vi "Actor Core.vi"(8 "error in":errorcluster, 11 "Commissioning in":refnum<class "Commissioning.lvclass">) -> (0 "error out":errorcluster, 3 "Actor out":refnum<class "Actor.lvclass">)   [LabVIEW 2018, in "Commissioning Actor.lvlib" / "Commissioning.lvclass"]
doc: "(<B>Filename</B>: Actor Framework.lvlib:Actor.lvclass:Actor Core.vi)\n\nReceives messages to the actor, reacts to them, and initiates any error handling that may shut the actor down.\n\nDescendant classes may override this VI to append parallel tasks for the actor to complete while it handles messages. Overrides use the Call Parent Method node."
uses:
  Commissioning.lvclass
  C:/Users/Administrator/Desktop/LabVIEW EMS/EMS Generic Actor/EMS Generic/EMS Generic.lvclass
  C:/Users/Administrator/Desktop/LabVIEW EMS/Device Communication and Control Abstract Actor/Device Communication and Control Abstract/Device Communication and Control Abstract.lvclass
  C:/Program Files (x86)/National Instruments/LabVIEW 2018/vi.lib/ActorFramework/Actor/Actor.lvclass
  <vilib>/ActorFramework/Actor/Actor.lvclass
  <vilib>/ORNL/CSEISMIC DDS/CSEISMIC DDS Base/Data Types/Controls/DeviceID.ctl
  EMS Generic Actor/EMS Generic/EMS Generic.lvclass/EMS Generic.ctl
  <vilib>/ORNL/CSEISMIC DDS/CSEISMIC DDS Base/Data Types/Controls/DeviceClass Selector.ctl
  <vilib>/ActorFramework/Actor/Actor.lvclass/Actor.ctl
  Device Communication and Control Abstract Actor/Device Communication and Control Abstract/Device Communication and Control Abstract.lvclass/Device Communication and Control Abstract.ctl
  <vilib>/ActorFramework/Message Enqueuer/Message Enqueuer.lvclass/Message Enqueuer.ctl
  Commissioning.lvclass/Commissioning.ctl
  Controls/Activate or Blackstart Selector.ctl
  Commissioning Messages/Activate or Blackstart Msg/Activate or Blackstart Msg.lvclass/Activate or Blackstart Msg.ctl
  <vilib>/ORNL/CSEISMIC DDS/CSEISMIC DDS Base/Data Types/DER_Measurement.ctl
  <vilib>/ORNL/CSEISMIC DDS/CSEISMIC DDS Base/Data Types/DER_Info.ctl
  <vilib>/ORNL/CSEISMIC DDS/CSEISMIC DDS Base/Data Types/Meter_Measurement.ctl
  <vilib>/ORNL/CSEISMIC DDS/CSEISMIC DDS Base/Data Types/Meter_Info.ctl
  <vilib>/ORNL/CSEISMIC DDS/CSEISMIC DDS Base/Data Types/SmartRelay_Measurement.ctl
  <vilib>/ORNL/CSEISMIC DDS/CSEISMIC DDS Base/Data Types/SmartRelay_Info.ctl
  <vilib>/ActorFramework/Message Enqueuer/Enqueue.vi
  EMS Generic Actor/EMS Generic/Accessors - Global Configuration/Read Global Configuration.vi
  Device Communication and Control Abstract Actor/Device Communication and Control Abstract Messages/Set IED MicrogridID Msg/Set IED MicrogridID Msg.lvclass
  C:/Program Files (x86)/National Instruments/LabVIEW 2018/vi.lib/ActorFramework/Message/Message.lvclass
  Commissioning Messages/Activate or Blackstart Msg/Activate or Blackstart Msg.lvclass
  <vilib>/ActorFramework/Message Priority Queue/Priority Enqueue.vi
  EMS Generic Actor/EMS Generic/Accessors - Global Configuration/Update Global Configuration.vi
  Generic Optimization Actor/Generic Optimization/Generic Optimization.lvclass
  Device Communication and Control Abstract Actor/Device Communication and Control Abstract/Device Communication and Control Abstract.lvclass
  EMS Generic Actor/EMS Generic/EMS Generic.lvclass
  <vilib>/ORNL/CSEISMIC DDS/CSEISMIC DDS Base/CSEISMIC DDS.lvclass
  Global Variables/Global Variables.vi
panel:
  out "PrimaryVoltage":dbl[](array[numeric])
  out "PCC DeviceID":T1
  out "Low Voltage":dbl
  out "High Voltage":dbl
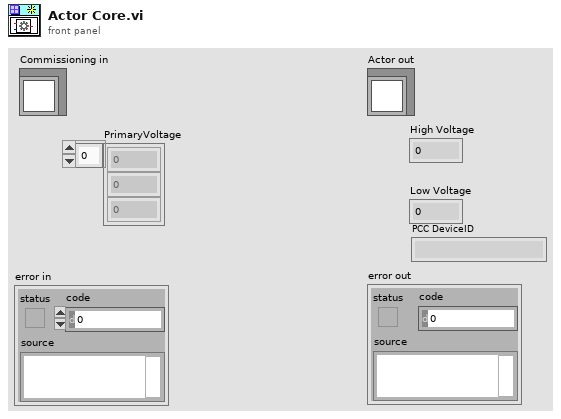
[diagram p1: front panel]
types:
  T1 = typedef "CSEISMIC DDS.lvlib/CSEISMIC DDS.lvclass/DeviceID.ctl" = string
  T2 = enum32{"Invalid", "Standard", "Closed", "Hidden", "Minimized", "Maximized"}
  T3 = typedef "EMS Generic Actor.lvlib/EMS Generic.lvclass/Data Type DVRs.ctl" = cluster{"IED_Status":refnum<data-value>, "IED_Status_0":refnum<data-value>, "DER_Measurement":refnum<data-value>, "DER_Info":refnum<data-value>, "DER_Status":refnum<data-value>, "ES_Measurement":refnum<data-value>, "ES_Info":refnum<data-value>, "PV_Info":refnum<data-value>, "SmartRelay_Info":refnum<data-value>, "SmartRelay_Measurement":refnum<data-value>, "Meter_Info":refnum<data-value>, "Meter_Measurement":refnum<data-value>, "HVAC_Status":refnum<data-value>, "HVAC_Measurement":refnum<data-value>, "PriceData_RealTime":refnum<data-value>, "PriceData_Demand":refnum<data-value>, "PriceData_Energy":refnum<data-value>, "ForecastData_Long":refnum<data-value>, "ForecastData_Short":refnum<data-value>, "DER_Control":refnum<data-value>, "DER_SetPointF":refnum<data-value>, "DER_SetPointP":refnum<data-value>, "DER_SetPointQ":refnum<data-value>, "DER_SetPointPF":refnum<data-value>, "DER_SetPointV":refnum<data-value>, "PV_setCurtailment":refnum<data-value>, "PV_setRampRate":refnum<data-value>, "Relay_Control":refnum<data-value>, "Load_Control":refnum<data-value>, "HVAC_Control":refnum<data-value>, "Generator_Info":refnum<data-value>, "ForecastData_Long_Backup":refnum<data-value>, "PriceData_RealTime_Backup":refnum<data-value>}
  T4 = typedef "CSEISMIC DDS.lvlib/CSEISMIC DDS.lvclass/DeviceClass Selector.ctl" = u16
  T5 = typedef "Commissioning Actor.lvlib/Commissioning.lvclass/Activate or Blackstart Selector.ctl" = enum16{"Activate", "Blackstart"}
  T6 = typedef "CSEISMIC DDS.lvlib/CSEISMIC DDS.lvclass/Meter_Info.ctl" = cluster{"DeviceID":T1, "LineConfig":u8[], "NominalVoltage(V)":dbl}
  T7 = typedef "CSEISMIC DDS.lvlib/CSEISMIC DDS.lvclass/Meter_Measurement.ctl" = cluster{"DeviceID":T1, "Voltage":dbl[], "Current":dbl[], "RealPower":dbl[], "ReactivePower":dbl[], "LineConfig":u8[], "Frequency":dbl}
  T8 = typedef "CSEISMIC DDS.lvlib/CSEISMIC DDS.lvclass/DER_Info.ctl" = cluster{"DeviceID":T1, "LineConfig":u8[], "NominalVoltage(V)":dbl, "PowerRating(kVA)":dbl, "VFControl":bool, "PControl":bool, "QControl":bool, "PFControl":bool, "PVControl":bool, "Droop":bool, "DroopConfigurable":bool, "Unbalanced":bool}
  T9 = typedef "CSEISMIC DDS.lvlib/CSEISMIC DDS.lvclass/DER_Measurement.ctl" = cluster{"DeviceID":T1, "Voltage":dbl[], "Current":dbl[], "RealPower":dbl[], "ReactivePower":dbl[], "LineConfig":u8[], "Frequency":dbl}
  T10 = typedef "CSEISMIC DDS.lvlib/CSEISMIC DDS.lvclass/SmartRelay_Info.ctl" = cluster{"DeviceID":T1, "LineConfig":u8[], "NominalVoltage(V)":dbl}
  T11 = typedef "CSEISMIC DDS.lvlib/CSEISMIC DDS.lvclass/SmartRelay_Measurement.ctl" = cluster{"DeviceID":T1, "PrimaryVoltage":dbl[], "SecondaryVoltage":dbl[], "Current":dbl[], "RealPower":dbl[], "ReactivePower":dbl[], "LineConfig":u8[], "Frequency":dbl}
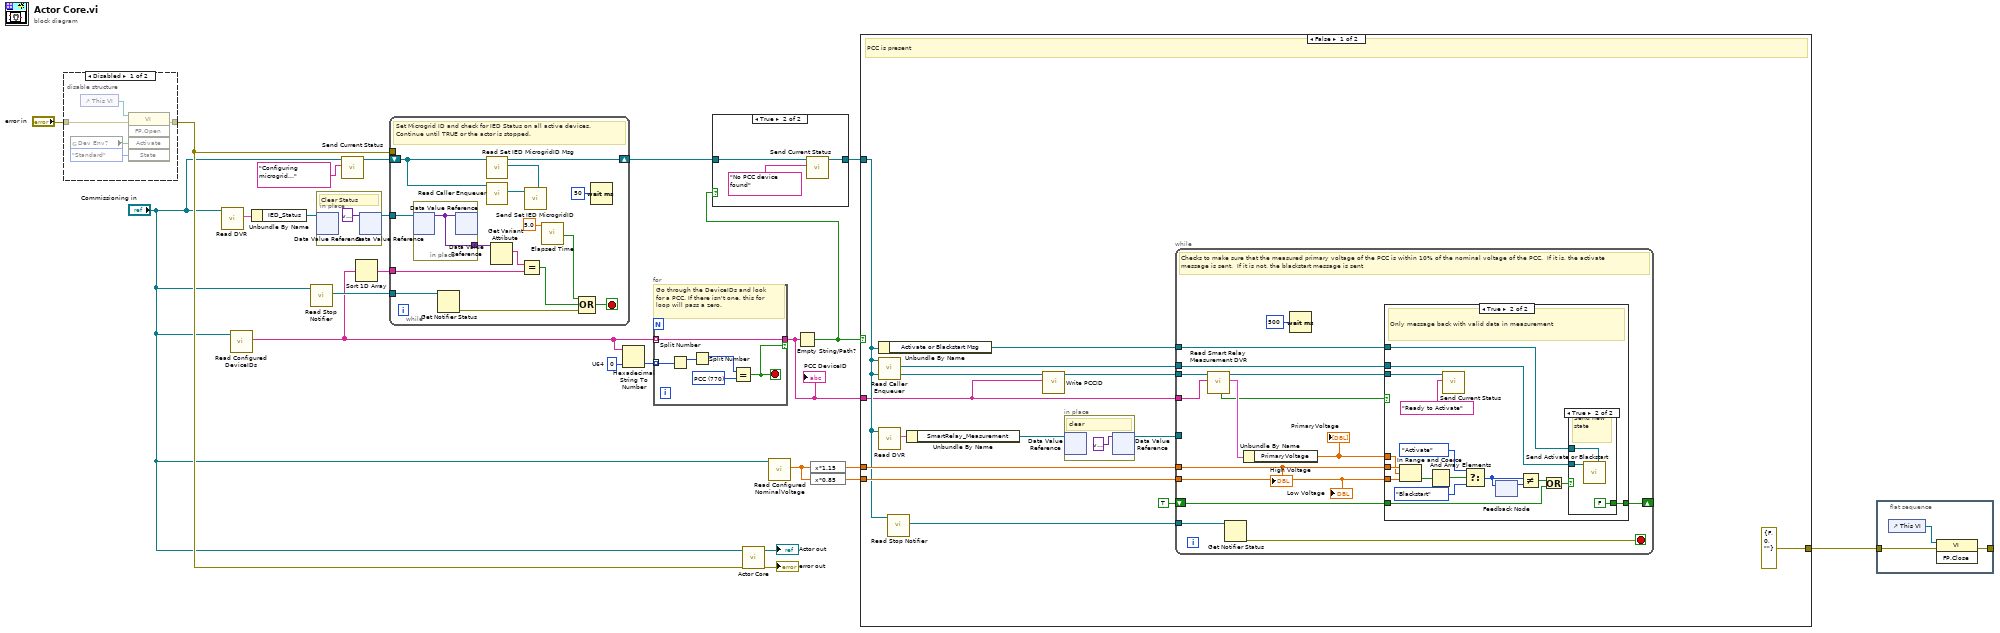
[diagram p0: block diagram]
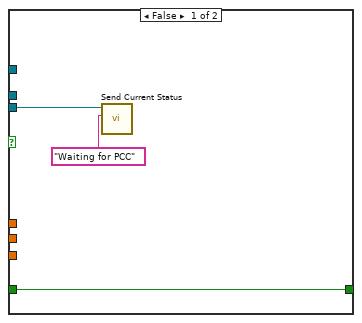
[diagram p4: hidden frame]
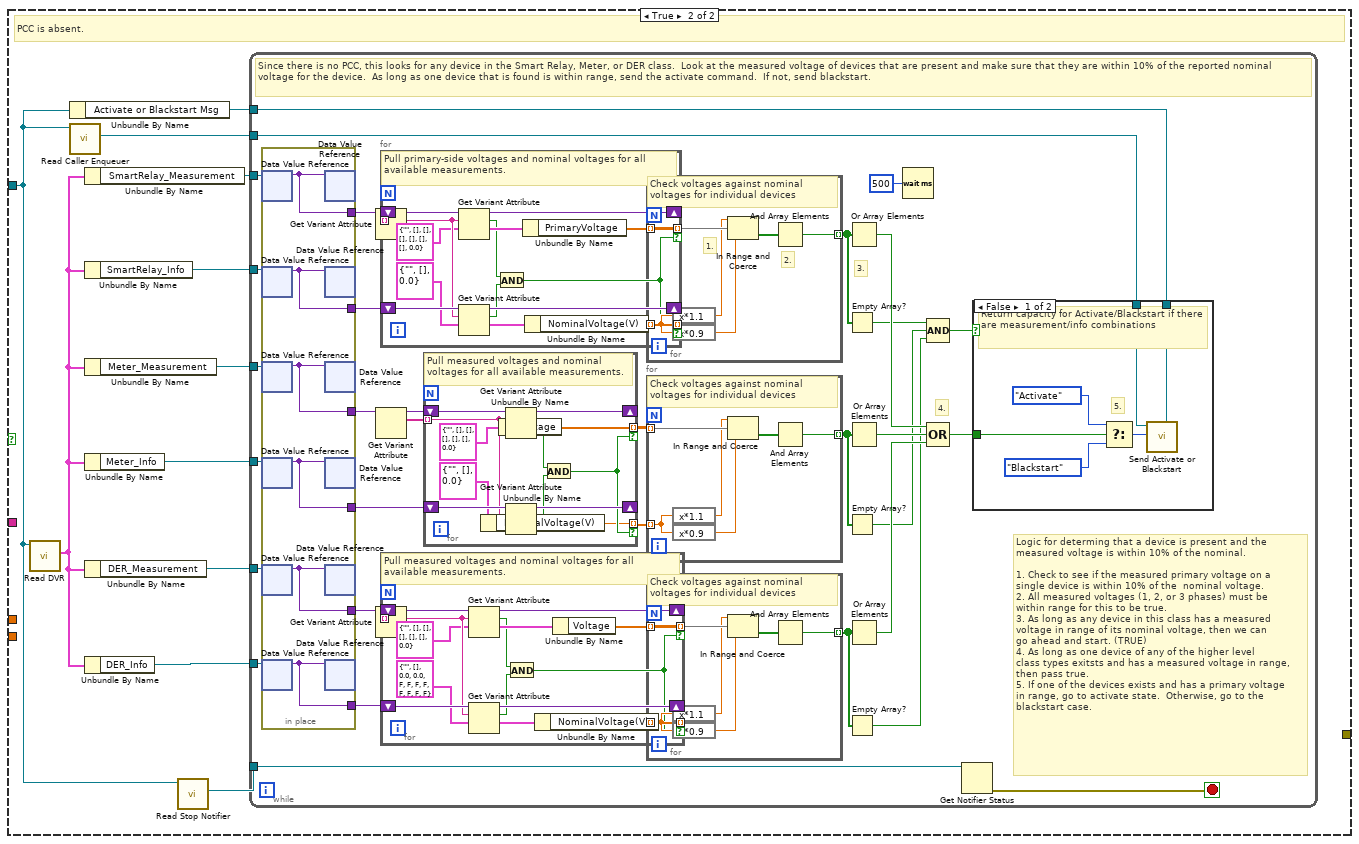
[diagram p6: hidden frame]
diagram:
  w15 = u64 0  # U64
  n1 = disable-structure shown="Disabled" {
    disable-tunnel: "error in" -> [w26 w29]
    disable-tunnel: [w25 w29] -> w10
    frame Disabled {
      n2 = global read "Global Variables.vi" "Dev Env?"() -> (w24:bool)
      n3 = control-ref of="This VI"() -> (w28:refnum<vi>)
      n4 = invoke class="VI" method="FP.Open"(reference=w28, error in=w26, "Activate"=w24, "State"=T2."Standard") -> (error out=w25:errorcluster)  [unwired: 1 in, 4 out]
    }
    frame Enabled {
    }
  }
  n5 = call "Read DVR.vi"("EMS Generic in"="Commissioning in") -> ("DVR"=w19:T3)  [unwired: 9 in, 1 out]
  n6 = call "Read Configured DeviceIDs.vi"("EMS Generic in"="Commissioning in") -> ("DeviceIDs"=w9:T1[])  [unwired: 8 in, 2 out]
  n7 = Unbundle By Name(w19) -> ("IED_Status"=w14:refnum<data-value>)
  n8 = call "Read Stop Notifier.vi"("EMS Generic in"="Commissioning in") -> ("stop"=w16:refnum<notifier>)  [unwired: 9 in, 1 out]
  n9 = in-place {
    # "Clear Status"
    n10 = in-place-dvr #1(w14) -> ()  [unwired: 2 out]
    n11 = in-place-dvr #1(variant ("data value")) -> (w13:refnum<data-value>)  [unwired: 1 out]
  }
  n12 = call "Send Current Status.vi"("Current Status"="Configuring microgrid...", "Device Communication and Control Abstract in"="Commissioning in") -> ("Device Communication and Control Abstract out"=w5:refnum<class "Commissioning.lvclass">)  [unwired: 8 in, 1 out]
  n13 = Sort 1D Array(array=w9) -> (sorted array=w8:T1[])
  n14 = while {
    tunnel: w13 -> [w41]
    tunnel: w16 -> [w45]
    shift-right: [w38] -> w3
    shift-left: w5 -> [w36]
    tunnel: w10 -> [_]
    tunnel: w8 -> [w33]
    stop <- w39 stop-if-true
    # "Set Microgrid ID and check for IED Status on all active devices. Continue until TRUE or the actor is stopped."
    n15 = in-place {
      in-place-border: [w46] -> w42
      n16 = in-place-dvr #2(w41) -> (w46:variant)  [unwired: 1 out]
      n17 = in-place-dvr #2(w46) -> ()  [unwired: 2 out]
    }
    n18 = Get Notifier Status(notifier=w45) -> (error out=w40:errorcluster)  [unwired: 1 in, 4 out]
    n19 = call "Read Set IED MicrogridID Msg.vi"("SCADA Sub Abstract in"=w36) -> ("Set IED MicrogridID Msg"=w43:refnum<class "Set IED MicrogridID Msg.lvclass">, "SCADA Sub Abstract out"=w38:refnum<class "Commissioning.lvclass">)  [unwired: 9 in]
    n20 = call <vilib>:"Read Caller Enqueuer.vi"("Actor"=w36) -> ("Caller Enqueuer"=w44:refnum<class "Message Enqueuer.lvclass">)  [unwired: 10 in]
    n21 = Get Variant Attribute(Variant=w42) -> (names=w35:string[])  [unwired: 3 in, 3 out]
    n22 = Equal?(x=w35, y=w33) -> (x = y?=w34:bool)
    n23 = call "Send Set IED MicrogridID.vi"("Message Type"=w43, "Message Enqueuer"=w44) -> ()  [unwired: 8 in, 2 out]
    n24 = call "Elapsed Time"("Time Target (s)"=5.0) -> ("Time has Elapsed"=w31:bool)  [unwired: 11 in, 7 out]
    n25 = Compound Arithmetic op=OR(w31, w34, w40) -> (w39:bool)
    n26 = Wait (ms)(milliseconds to wait=u32 50) -> ()  [unwired: 1 out]
  }
  n27 = Hexadecimal String To Number(string=w9, default (0uL)=w15) -> (number=w18:u64[])  [unwired: 1 in, 1 out]
  n28 = for {
    tunnel: w9 -> [w51] mode=indexing
    tunnel: [w51] -> w22 if=w48
    tunnel: w18 -> [w47] mode=indexing
    stop <- w48 stop-if-true
    w50 = T4 770 items=["Invalid"=0, "IED"=256, "DER"=512, "Relay"=768, "Meter"=1024, "Load"=1280, "Energy Storage"=513, "PV"=514, "Generator"=515, "Smart Relay"=769, "PCC"=770, "Smart Meter"=1025, "PMU"=1026, "HVAC"=1281] ("DeviceClass")
    # "Go through the DeviceIDs and look for a PCC. If there isn't one, this for loop will pass a zero."
    n29 = Split Number(x=w47) -> (hi(x)=w52:u32)  [unwired: 1 out]
    n30 = Split Number(x=w52) -> (hi(x)=w49:u16)  [unwired: 1 out]
    n31 = Equal?(x=w49, y=w50) -> (x = y?=w48:bool)
  }
  "PCC DeviceID" <- w22
  n32 = call-parent "Actor Core.vi"("error in"=w10, "Actor in"="Commissioning in") -> ("error out"=→"error out":errorcluster, "Actor out"=→"Actor out":refnum<class "Actor.lvclass">)  [unwired: 8 in]
  n33 = call "Read Configured NominalVoltage.vi"("EMS Generic in"="Commissioning in") -> ("NominalVoltage"=w7:dbl)  [unwired: 8 in, 2 out]
  n34 = Empty String/Path?(string/path=w22) -> (empty?=w1:bool)
  n35 = case shown="True" w1 {
    tunnel: w3 -> [w53 w55]
    tunnel: [w53 w54] -> w2
    frame False {
    }
    frame True {
      n36 = call "Send Current Status.vi"("Current Status"="No PCC device found", "Device Communication and Control Abstract in"=w55) -> ("Device Communication and Control Abstract out"=w54:refnum<class "Commissioning.lvclass">)  [unwired: 8 in, 1 out]
    }
  }
  n37 = expression code="x*1.15"(w7) -> (w21:dbl)
  n38 = expression code="x*0.85"(w7) -> (w20:dbl)
  n39 = case shown="False" w1 {
    tunnel: w22 -> [w59 _]
    tunnel: w2 -> [w60 w109]
    tunnel: w21 -> [w68 _]
    tunnel: w20 -> [w67 _]
    tunnel: [errorcluster {"status"=FALSE, "code"=0, "source"=""} ("error in (no error)") _] -> w12
    frame False {
      # "PCC is present"
      n40 = Unbundle By Name(w60) -> ("Activate or Blackstart Msg"=w65:refnum<class "Activate or Blackstart Msg.lvclass">)
      n41 = call <vilib>:"Read Caller Enqueuer.vi"("Actor"=w60) -> ("Caller Enqueuer"=w66:refnum<class "Message Enqueuer.lvclass">)  [unwired: 10 in]
      n42 = call "Read DVR.vi"("EMS Generic in"=w60) -> ("DVR"=w69:T3)  [unwired: 9 in, 1 out]
      n43 = call "Read Stop Notifier.vi"("EMS Generic in"=w60) -> ("stop"=w64:refnum<notifier>)  [unwired: 9 in, 1 out]
      n44 = Unbundle By Name(w69) -> ("SmartRelay_Measurement"=w63:refnum<data-value>)
      n45 = call "Write PCCID.vi"("PCCID"=w59, "EMS Generic in"=w60) -> ("EMS Generic out"=w58:refnum<class "Commissioning.lvclass">)  [unwired: 8 in, 1 out]
      n46 = in-place {
        # "clear"
        n47 = in-place-dvr #3(w63) -> ()  [unwired: 2 out]
        n48 = in-place-dvr #3(variant ("data value")) -> (w62:refnum<data-value>)  [unwired: 1 out]
      }
      n49 = while {
        tunnel: w62 -> [_]
        tunnel: w59 -> [w76]
        tunnel: w68 -> [w85]
        tunnel: w67 -> [w84]
        tunnel: w66 -> [w82]
        tunnel: w65 -> [w81]
        tunnel: w64 -> [w80]
        tunnel: w58 -> [w77]
        shift-right: [w71] -> _
        shift-left: TRUE -> [w72]
        stop <- w79 stop-if-true
        # "Checks to make sure that the measured primary voltage of the PCC is within 10% of the nominal voltage of the PCC.  If it is, the activate message is sent.  If it is not, the blackstart message is sent"
        n50 = call "Read Smart Relay Measurement DVR.vi"("DeviceID"=w76, "EMS Generic in"=w77) -> ("SmartRelay_Measurement"=w75:T11, "EMS Generic out"=w73:refnum<class "Commissioning.lvclass">, "valid?"=w74:bool)  [unwired: 6 in, 1 out]
        n51 = Get Notifier Status(notifier=w80) -> (error out=w79:errorcluster)  [unwired: 1 in, 4 out]
        n52 = Unbundle By Name(w75) -> ("PrimaryVoltage"=w83:dbl[])
        "PrimaryVoltage" <- w83
        n53 = Wait (ms)(milliseconds to wait=u32 500) -> ()  [unwired: 1 out]
        n54 = case shown="True" w74 {
          tunnel: w85 -> [_ w105]
          tunnel: w84 -> [_ w104]
          tunnel: w83 -> [_ w103]
          tunnel: w82 -> [_ w101]
          tunnel: w81 -> [_ w100]
          tunnel: w73 -> [w87 w95]
          tunnel: w72 -> [w86 w90]
          tunnel: [w86 w89] -> w71
          frame False {
            n55 = call "Send Current Status.vi"("Current Status"="Waiting for PCC", "Device Communication and Control Abstract in"=w87) -> ()  [unwired: 8 in, 2 out]
          }
          frame True {
            # "Only message back with valid data in measurement"
            n56 = In Range and Coerce(upper limit=w105, x=w103, lower limit=w104) -> (In Range?=w102:bool[])  [unwired: 1 out]
            n57 = And Array Elements(Boolean array=w102) -> (logical AND=w99:bool)
            n58 = call "Send Current Status.vi"("Current Status"="Ready to Activate", "Device Communication and Control Abstract in"=w95) -> ()  [unwired: 8 in, 2 out]
            n59 = Select(t=Activate_or_Blackstart_Selector."Activate" ("Activate or Blackstart"), s=w99, f=Activate_or_Blackstart_Selector."Blackstart" ("Activate or Blackstart")) -> (s? t:f=w93:T5)
            n60 = feedback-in #4(w93) -> ()
            n61 = feedback #4() -> (w94:T5)  [unwired: 1 in]
            n62 = Not Equal?(x=w93, y=w94) -> (x != y?=w92:bool)
            n63 = Or(x=w92, y=w90) -> (x .or. y?=w91:bool)
            n64 = case shown="True" w91 {
              tunnel: w101 -> [_ w108]
              tunnel: w100 -> [_ w107]
              tunnel: [_ FALSE] -> w89
              frame False {
                # "Already sent this message.  Do nothing."
              }
              frame True {
                # "Send new state"
                n65 = call "Send Activate or Blackstart.vi"("Message Type"=w107, "Message Enqueuer"=w108) -> ()  [unwired: 8 in, 2 out]
              }
            }
          }
        }
        "High Voltage" <- w85
        "Low Voltage" <- w84
      }
    }
    frame True {
      # "PCC is absent."
      n66 = call "Read DVR.vi"("EMS Generic in"=w109) -> ("DVR"=w111:T3)  [unwired: 9 in, 1 out]
      n67 = Unbundle By Name(w109) -> ("Activate or Blackstart Msg"=w113:refnum<class "Activate or Blackstart Msg.lvclass">)
      n68 = call <vilib>:"Read Caller Enqueuer.vi"("Actor"=w109) -> ("Caller Enqueuer"=w112:refnum<class "Message Enqueuer.lvclass">)  [unwired: 10 in]
      n69 = Unbundle By Name(w111) -> ("SmartRelay_Measurement"=w114:refnum<data-value>)
      n70 = Unbundle By Name(w111) -> ("SmartRelay_Info"=w115:refnum<data-value>)
      n71 = Unbundle By Name(w111) -> ("Meter_Measurement"=w116:refnum<data-value>)
      n72 = Unbundle By Name(w111) -> ("Meter_Info"=w118:refnum<data-value>)
      n73 = Unbundle By Name(w111) -> ("DER_Measurement"=w117:refnum<data-value>)
      n74 = Unbundle By Name(w111) -> ("DER_Info"=w119:refnum<data-value>)
      n75 = call "Read Stop Notifier.vi"("EMS Generic in"=w109) -> ("stop"=w110:refnum<notifier>)  [unwired: 9 in, 1 out]
      n76 = while {
        tunnel: w119 -> [w159]
        tunnel: w118 -> [w158]
        tunnel: w117 -> [w157]
        tunnel: w116 -> [w156]
        tunnel: w115 -> [w155]
        tunnel: w114 -> [w154]
        tunnel: w113 -> [w131]
        tunnel: w112 -> [w121]
        tunnel: w110 -> [w130]
        stop <- w129 stop-if-true
        # "Logic for determing that a device is present and the\nmeasured voltage is within 10% of the nominal.\n\n1. Check to see if the measured primary voltage on a\nsingle device is within 10% of the  nominal voltage.\n2. All measured voltages (1, 2, or 3 phases) must be \nwithin range for this to be true.\n3. As long as any device in this class has a measured\nvoltage in range of its nominal voltage, then we can\ngo ahead and start. (TRUE)\n4. As long as one device of any of the higher level \nclass types exitsts and has a measured voltage in range,\nthen pass true.\n5. If one of the devices exists and has a primary voltage\nin range, go to activate state.  Otherwise, go to the\nblackstart case."
        # "4."
        # "3."
        # "Since there is no PCC, this looks for any device in the Smart Relay, Meter, or DER class.  Look at the measured voltage of devices that are present and make sure that they are within 10% of the reported nominal voltage for the device.  As long as one device that is found is within range, send the activate command.  If not, send blackstart."
        n77 = in-place {
          in-place-border: [w179] -> w151
          in-place-border: [w178] -> w150
          in-place-border: [w177] -> w147
          in-place-border: [w176] -> w146
          in-place-border: [w175] -> w143
          in-place-border: [w174] -> w142
          n78 = in-place-dvr #5(w154) -> (w179:variant)  [unwired: 1 out]
          n79 = in-place-dvr #6(w155) -> (w178:variant)  [unwired: 1 out]
          n80 = in-place-dvr #7(w156) -> (w177:variant)  [unwired: 1 out]
          n81 = in-place-dvr #8(w158) -> (w176:variant)  [unwired: 1 out]
          n82 = in-place-dvr #9(w157) -> (w175:variant)  [unwired: 1 out]
          n83 = in-place-dvr #10(w159) -> (w174:variant)  [unwired: 1 out]
          n84 = in-place-dvr #5(w179) -> ()  [unwired: 2 out]
          n85 = in-place-dvr #6(w178) -> ()  [unwired: 2 out]
          n86 = in-place-dvr #7(w177) -> ()  [unwired: 2 out]
          n87 = in-place-dvr #8(w176) -> ()  [unwired: 2 out]
          n88 = in-place-dvr #9(w175) -> ()  [unwired: 2 out]
          n89 = in-place-dvr #10(w174) -> ()  [unwired: 2 out]
        }
        n90 = Get Variant Attribute(Variant=w151) -> (duplicate Variant=w152:variant, names=w153:string[])  [unwired: 3 in, 2 out]
        n91 = Get Variant Attribute(Variant=w147) -> (duplicate Variant=w149:variant, names=w148:string[])  [unwired: 3 in, 2 out]
        n92 = Get Variant Attribute(Variant=w143) -> (duplicate Variant=w144:variant, names=w145:string[])  [unwired: 3 in, 2 out]
        n93 = for {
          shift-right: [w206] -> _
          shift-left: w152 -> [w207]
          shift-right: [w204] -> _
          shift-left: w150 -> [w205]
          tunnel: w153 -> [w203] mode=indexing
          tunnel: [w195] -> w140 mode=indexing if=w196
          tunnel: [w194] -> w141 mode=indexing if=w196
          # "Pull primary-side voltages and nominal voltages for all available measurements."
          n94 = Get Variant Attribute(Variant=w207, name=w203, default value (empty Variant)=T11 {"DeviceID"="", "PrimaryVoltage"=[], "SecondaryVoltage"=[], "Current"=[], "RealPower"=[], "ReactivePower"=[], "LineConfig"=[], "Frequency"=0.0} ("SmartRelay_Measurement")) -> (duplicate Variant=w206:variant, found=w199:bool, value=w201:T11)  [unwired: 1 in, 1 out]
          n95 = Get Variant Attribute(Variant=w205, name=w203, default value (empty Variant)=T10 {"DeviceID"="", "LineConfig"=[], "NominalVoltage(V)"=0.0} ("SmartRelay_Info")) -> (duplicate Variant=w204:variant, found=w200:bool, value=w197:T10)  [unwired: 1 in, 1 out]
          n96 = And(x=w199, y=w200) -> (x .and. y?=w196:bool)
          n97 = Unbundle By Name(w201) -> ("PrimaryVoltage"=w195:dbl[])
          n98 = Unbundle By Name(w197) -> ("NominalVoltage(V)"=w194:dbl)
        }
        n99 = for {
          shift-right: [w192] -> _
          shift-left: w144 -> [w193]
          shift-right: [w190] -> _
          shift-left: w142 -> [w191]
          tunnel: w145 -> [w189] mode=indexing
          tunnel: [w183] -> w138 mode=indexing if=w184
          tunnel: [w182] -> w137 mode=indexing if=w184
          # "Pull measured voltages and nominal voltages for all available measurements."
          n100 = Get Variant Attribute(Variant=w193, name=w189, default value (empty Variant)=T9 {"DeviceID"="", "Voltage"=[], "Current"=[], "RealPower"=[], "ReactivePower"=[], "LineConfig"=[], "Frequency"=0.0} ("DER_Measurement")) -> (duplicate Variant=w192:variant, found=w186:bool, value=w188:T9)  [unwired: 1 in, 1 out]
          n101 = Get Variant Attribute(Variant=w191, name=w189, default value (empty Variant)=T8 {"DeviceID"="", "LineConfig"=[], "NominalVoltage(V)"=0.0, "PowerRating(kVA)"=0.0, "VFControl"=FALSE, "PControl"=FALSE, "QControl"=FALSE, "PFControl"=FALSE, "PVControl"=FALSE, "Droop"=FALSE, "DroopConfigurable"=FALSE, "Unbalanced"=FALSE} ("DER_Info")) -> (duplicate Variant=w190:variant, found=w187:bool, value=w185:T8)  [unwired: 1 in, 1 out]
          n102 = And(x=w186, y=w187) -> (x .and. y?=w184:bool)
          n103 = Unbundle By Name(w185) -> ("NominalVoltage(V)"=w182:dbl)
          n104 = Unbundle By Name(w188) -> ("Voltage"=w183:dbl[])
        }
        n105 = for {
          shift-right: [w172] -> _
          shift-left: w149 -> [w173]
          shift-right: [w170] -> _
          shift-left: w146 -> [w171]
          tunnel: w148 -> [w169] mode=indexing
          tunnel: [w163] -> w139 mode=indexing if=w164
          tunnel: [w162] -> w136 mode=indexing if=w164
          # "Pull measured voltages and nominal voltages for all available measurements."
          n106 = Get Variant Attribute(Variant=w173, name=w169, default value (empty Variant)=T7 {"DeviceID"="", "Voltage"=[], "Current"=[], "RealPower"=[], "ReactivePower"=[], "LineConfig"=[], "Frequency"=0.0} ("Meter_Measurement")) -> (duplicate Variant=w172:variant, found=w166:bool, value=w168:T7)  [unwired: 1 in, 1 out]
          n107 = Unbundle By Name(w168) -> ("Voltage"=w163:dbl[])
          n108 = Get Variant Attribute(Variant=w171, name=w169, default value (empty Variant)=T6 {"DeviceID"="", "LineConfig"=[], "NominalVoltage(V)"=0.0} ("Meter_Info")) -> (duplicate Variant=w170:variant, found=w167:bool, value=w165:T6)  [unwired: 1 in, 1 out]
          n109 = Unbundle By Name(w165) -> ("NominalVoltage(V)"=w162:dbl)
          n110 = And(x=w166, y=w167) -> (x .and. y?=w164:bool)
        }
        n111 = for {
          tunnel: w141 -> [w231] mode=indexing
          tunnel: w140 -> [w230] mode=indexing
          tunnel: [w226] -> w127 mode=indexing
          # "2."
          # "1."
          # "Check voltages against nominal voltages for individual devices"
          n112 = expression code="x*1.1"(w231) -> (w229:dbl)
          n113 = expression code="x*0.9"(w231) -> (w228:dbl)
          n114 = In Range and Coerce(upper limit=w229, x=w230, lower limit=w228) -> (In Range?=w227:bool[])  [unwired: 1 out]
          n115 = And Array Elements(Boolean array=w227) -> (logical AND=w226:bool)
        }
        n116 = for {
          tunnel: w136 -> [w225] mode=indexing
          tunnel: w139 -> [w224] mode=indexing
          tunnel: [w220] -> w126 mode=indexing
          # "Check voltages against nominal voltages for individual devices"
          n117 = expression code="x*1.1"(w225) -> (w223:dbl)
          n118 = expression code="x*0.9"(w225) -> (w222:dbl)
          n119 = In Range and Coerce(upper limit=w223, x=w224, lower limit=w222) -> (In Range?=w221:bool[])  [unwired: 1 out]
          n120 = And Array Elements(Boolean array=w221) -> (logical AND=w220:bool)
        }
        n121 = for {
          tunnel: w137 -> [w219] mode=indexing
          tunnel: w138 -> [w218] mode=indexing
          tunnel: [w214] -> w125 mode=indexing
          # "Check voltages against nominal voltages for individual devices"
          n122 = expression code="x*1.1"(w219) -> (w217:dbl)
          n123 = expression code="x*0.9"(w219) -> (w216:dbl)
          n124 = In Range and Coerce(upper limit=w217, x=w218, lower limit=w216) -> (In Range?=w215:bool[])  [unwired: 1 out]
          n125 = And Array Elements(Boolean array=w215) -> (logical AND=w214:bool)
        }
        n126 = Empty Array?(array=w127) -> (empty?=w124:bool)
        n127 = Empty Array?(array=w126) -> (empty?=w123:bool)
        n128 = Empty Array?(array=w125) -> (empty?=w122:bool)
        n129 = Or Array Elements(Boolean array=w127) -> (logical OR=w135:bool)
        n130 = Or Array Elements(Boolean array=w126) -> (logical OR=w134:bool)
        n131 = Or Array Elements(Boolean array=w125) -> (logical OR=w133:bool)
        n132 = Wait (ms)(milliseconds to wait=u32 500) -> ()  [unwired: 1 out]
        n133 = Compound Arithmetic op=AND(w124, w123, w122) -> (w120:bool)
        n134 = Compound Arithmetic op=OR(w135, w134, w133) -> (w132:bool)
        n135 = Get Notifier Status(notifier=w130) -> (error out=w129:errorcluster)  [unwired: 1 in, 4 out]
        n136 = case shown="False" w120 {
          tunnel: w132 -> [w210 _]
          tunnel: w131 -> [w209 _]
          tunnel: w121 -> [w208 _]
          frame False {
            # "5."
            # "Return capacity for Activate/Blackstart if there are measurement/info combinations"
            n137 = Select(t=Activate_or_Blackstart_Selector."Activate" ("Activate or Blackstart"), s=w210, f=Activate_or_Blackstart_Selector."Blackstart" ("Activate or Blackstart")) -> (s? t:f=w213:T5)
            n138 = call "Send Activate or Blackstart.vi"("Message Type"=w209, "Activate or Blackstart"=w213, "Message Enqueuer"=w208) -> ()  [unwired: 7 in, 2 out]
          }
          frame True {
          }
        }
      }
    }
  }
  n139 = flat-sequence {
    tunnel: w12 -> [w233]
    tunnel: [w232] -> _
    frame #0 {
      n140 = control-ref of="This VI"() -> (w234:refnum<vi>)
      n141 = invoke class="VI" method="FP.Close"(reference=w234, error in=w233) -> (error out=w232:errorcluster)  [unwired: 1 in, 2 out]
    }
  }
